vi "destroy.vi"(8 "error in (no error)":errorcluster, 11 "manager_daemon in":refnum<class "manager_daemon.lvclass">) -> (0 "error out":errorcluster, 3 "manager_daemon out":refnum<class "manager_daemon.lvclass">)   [LabVIEW 2024, in "manager_daemon.lvclass"]
uses:
  manager_daemon.lvclass
  type_defs/msg--cluster.ctl
  type_defs/cmd--enum.ctl
  manager_daemon.lvclass/manager_daemon.ctl
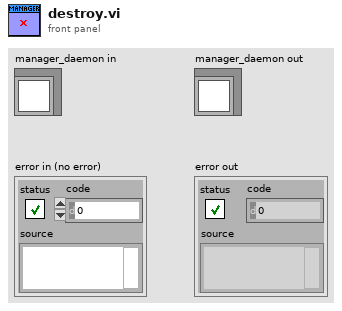
[diagram p1: front panel]
types:
  T1 = typedef "manager_daemon.lvclass/msg--cluster.ctl" = cluster{"cmd":T2, "data":variant}
  T2 = typedef "manager_daemon.lvclass/cmd--enum.ctl" = enum16{"init", "run", "load binaries", "build binaries", "save binaries", "updated volume", "return vol path by id", "return vol ids by publisher", "display info", "filter release week", "apply filter", "add publisher", "get publishers", "add volume", "add issues", "add issue", "delete volume", "delete issues", "download issues", "exit"}
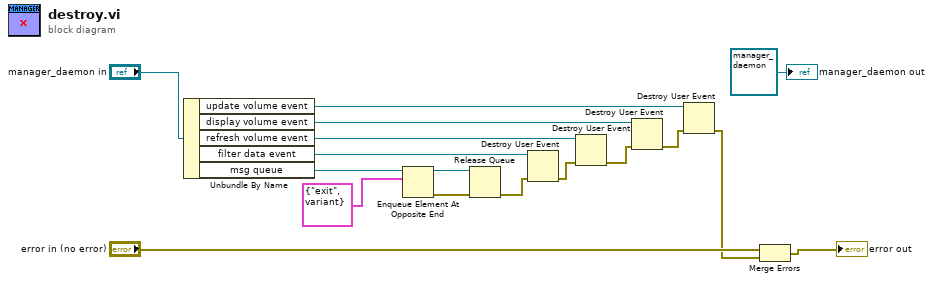
[diagram p0: block diagram]
diagram:
  n1 = Unbundle By Name("manager_daemon in") -> ("update volume event"=w6:refnum<user-event>, "display volume event"=w7:refnum<user-event>, "refresh volume event"=w8:refnum<user-event>, "filter data event"=w9:refnum<user-event>, "msg queue"=w15:refnum<queue>)
  n2 = Enqueue Element At Opposite End(queue=w15, element=T1 {"cmd"=enum."exit", "data"=variant}) -> (queue out=w13:refnum<queue>, error out=w12:errorcluster)  [unwired: 2 in, 1 out]
  n3 = Release Queue(queue=w13, error in (no error)=w12) -> (error out=w5:errorcluster)  [unwired: 1 in, 2 out]
  n4 = Destroy User Event(user event=w9, error in=w5) -> (error out=w4:errorcluster)
  n5 = Destroy User Event(user event=w8, error in=w4) -> (error out=w3:errorcluster)
  n6 = Destroy User Event(user event=w7, error in=w3) -> (error out=w2:errorcluster)
  n7 = Destroy User Event(user event=w6, error in=w2) -> (error out=w1:errorcluster)
  n8 = Merge Errors("error in (no error)", w1) -> (→"error out":errorcluster)
  "manager_daemon out" <- refnum<class "manager_daemon.lvclass"> refnum ("manager_daemon out")
